vi "Sine Integral.vi"(3 "x":dbl format="%.2f") -> (1 "Si(x)":dbl format="%.2f")   [LabVIEW 2020, in "NI_Gmath.lvlib"]
doc: "Evaluates the sine integral for any real number <B>x</B>."
uses:
  <vilib>/gmath/NI_Gmath.lvlib
  <resource>/lvanlys.dll
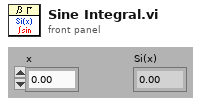
[diagram p1: front panel]
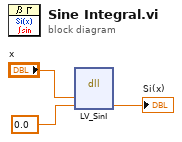
[diagram p0: block diagram]
diagram:
  n1 = dll-call lib="e:/builds/penguin/labview/branches/2020/dev/dist/resource/lvanlys.*" fn="LV_SinI"("x"="x", "SinI(x)"=0.0 ("cosI")) -> ("SinI(x)"=→"Si(x)":dbl)  [unwired: 5 in, 2 out]
